vi "roulette stand.vi"() -> ()   [LabVIEW 2019]
uses:
  <vilib>/Rock Robotics/WPI/ThirdParty/Phoenix-LabVIEW/Motor Controller/Controls/CTRE_Phoenix_MotorControl_ControlMode.ctl
panel:
  in  "up":bool
  in  "stand":bool
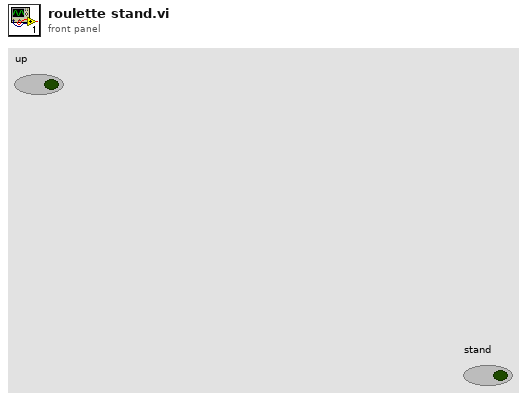
[diagram p1: front panel]
types:
  T1 = typedef "WPI_JoystickDevRef.ctl" = cluster{"Device":T2}
  T2 = typedef "WPI_JoystickDeviceEnum.ctl" = enum16{"USB 0", "USB 1", "USB 2", "USB 3", "USB 4", "USB 5"}
  T3 = typedef "WPI_MotorControlDeviceRef.ctl" = cluster{"DeviceStatus":errorcluster, "Type":T4, "PWM":cluster{"PWM Channel":T5, "DeadBand":T6}, "CAN":cluster{"Device Number":u8, "SetOutput VI Ref":variant, "GetOutput VI Ref":variant, "Enable VI Ref":variant, "Disable VI Ref":variant, "Data":variant}, "Invert":bool, "DIO PWM":cluster{"PWM \"Enable\" Channel":T5, "DIOChannel":T7, "PWM Rate":dbl}}
  T4 = typedef "WPI_MotorControlType.ctl" = enum16{"PWM", "CAN", "DIO PWM"}
  T5 = typedef "FPGA_DIOPWMChannel.ctl" = enum8{"PWM 0", "PWM 1", "PWM 2", "PWM 3", "PWM 4", "PWM 5", "PWM 6", "PWM 7", "PWM 8", "PWM 9", "PWM MXP 0", "PWM MXP 1", "PWM MXP 2", "PWM MXP 3", "PWM MXP 4", "PWM MXP 5", "PWM MXP 6", "PWM MXP 7", "PWM MXP 8", "PWM MXP 9", "Invalid"}
  T6 = typedef "WPI_PWMDeadband.ctl" = cluster{"Name":string, "maxPositivePwm":i32, "minPositivePwm":i32, "centerPwm":i32, "maxNegativePwm":i32, "minNegativePwm":i32, "angularRange":u16}
  T7 = typedef "FPGA_DIOChannel.ctl" = enum8{"DIO 0", "DIO 1", "DIO 2", "DIO 3", "DIO 4", "DIO 5", "DIO 6", "DIO 7", "DIO 8", "DIO 9", "DIO MXP 0", "DIO MXP 1", "DIO MXP 2", "DIO MXP 3", "DIO MXP 4", "DIO MXP 5", "DIO MXP 6", "DIO MXP 7", "DIO MXP 8", "DIO MXP 9", "DIO MXP 10", "DIO MXP 11", "DIO MXP 12", "DIO MXP 13", "DIO MXP 14", "DIO MXP 15", "SPI Port CS1", "SPI Port CS2", "SPI Port CS3", "SPI Port MISO", "SPI Port MOSI", "Invalid"}
  T8 = typedef "CTRE_Phoenix_MotorControl_ControlMode.ctl" = u16
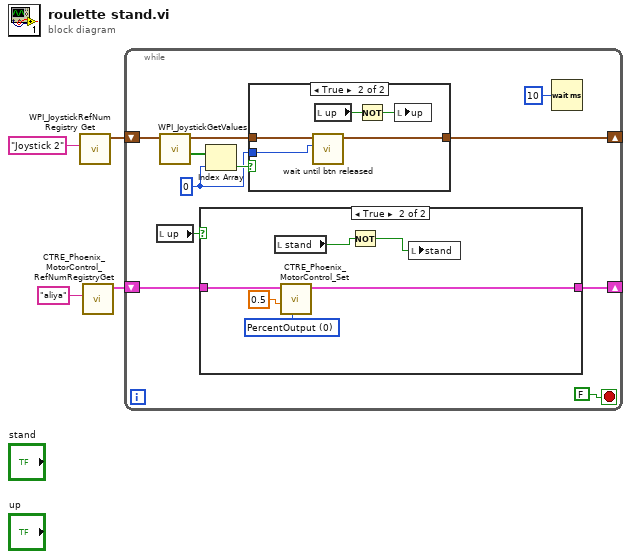
[diagram p0: block diagram]
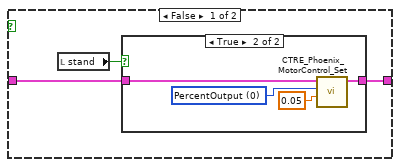
[diagram p2: hidden frame]
diagram:
  n1 = call <vilib>:"WPI_JoystickRefNum Registry Get.vi"("refnum name"="Joystick 2") -> ("JoystickDevRef"=w4:T1)  [unwired: 9 in, 1 out]
  n2 = call <vilib>:"CTRE_Phoenix_MotorControl_RefNumRegistryGet.vi"("refnum name"="aliya") -> ("PhoenixMotorControlDevRef"=w1:T3)  [unwired: 9 in, 1 out]
  n3 = while {
    shift-right: [w6] -> _
    shift-left: w1 -> [w7]
    shift-right: [w9] -> _
    shift-left: w4 -> [w15]
    stop <- FALSE stop-if-true
    w11 = 0 ("index")
    n4 = local read "up"() -> (w8:bool)
    n5 = call <vilib>:"WPI_JoystickGetValues.vi"("JoystickDevRef"=w15) -> ("Buttons"=w14:bool[], "JoystickDevRef"=w12:T1)  [unwired: 6 in, 3 out]
    n6 = case shown="True" w8 {
      tunnel: [w17 w29] -> w6
      tunnel: w7 -> [w16 w28]
      frame False {
        n7 = local read "stand"() -> (w18:bool)
        n8 = case shown="True" w18 {
          tunnel: w16 -> [w19 w23]
          tunnel: [w19 w22] -> w17
          frame False {
          }
          frame True {
            w20 = T8 0 items=["PercentOutput"=0, "Position"=1, "Velocity"=2, "Current"=3, "Follower"=5, "MotionProfile"=6, "MotionMagic"=7, "MotionProfileArc"=10, "Disabled"=15] ("Control Mode")
            n9 = call <vilib>:"CTRE_Phoenix_MotorControl_Set.vi"("Output"=0.05, "Control Mode"=w20, "PhoenixMotorControlDevRef"=w23) -> ("PhoenixMotorControlDevRef"=w22:T3)  [unwired: 7 in, 1 out]
          }
        }
      }
      frame True {
        w24 = T8 0 items=["PercentOutput"=0, "Position"=1, "Velocity"=2, "Current"=3, "Follower"=5, "MotionProfile"=6, "MotionMagic"=7, "MotionProfileArc"=10, "Disabled"=15] ("Control Mode")
        n10 = local read "stand"() -> (w26:bool)
        n11 = call <vilib>:"CTRE_Phoenix_MotorControl_Set.vi"("Output"=0.5, "Control Mode"=w24, "PhoenixMotorControlDevRef"=w28) -> ("PhoenixMotorControlDevRef"=w29:T3)  [unwired: 7 in, 1 out]
        n12 = Not(x=w26) -> (.not. x?=w25:bool)
        n13 = local write "stand"(w25) -> ()
      }
    }
    n14 = Index Array(array=w14, index=w11) -> (element=w13:bool)
    n15 = case shown="True" w13 {
      tunnel: w12 -> [w30 w32]
      tunnel: [w30 w33] -> w9
      tunnel: w11 -> [_ w31]
      frame False {
      }
      frame True {
        n16 = call "wait until btn released.vi"("index"=w31, "JoystickDevRef"=w32) -> ("JoystickDevRef 2"=w33:T1)  [unwired: 9 in]
        n17 = local read "up"() -> (w35:bool)
        n18 = Not(x=w35) -> (.not. x?=w34:bool)
        n19 = local write "up"(w34) -> ()
      }
    }
    n20 = Wait (ms)(milliseconds to wait=u32 10) -> ()  [unwired: 1 out]
  }
